vi "DB Message Loop.vi"(8 "error in (no error)":errorcluster, 11 "Message Queues":T1) -> (0 "error out":errorcluster)   [LabVIEW 2026]
uses:
  support/Message Queue/All Message Queues.ctl
  support/Message Queue/Message Cluster.ctl
  <vilib>/addons/database/Connection.llb/Conn ObjectReference.ctl
  controls/Telemetry_Data_Type.ctl
  controls/Channels.ctl
  controls/Error_Payload.ctl
  <vilib>/addons/database/Connection.llb/DB Tools Open Connec (String).vi
  <vilib>/addons/database/Connection.llb/Conn Execute.vi
  <vilib>/addons/database/Recordset.llb/Rec Destroy - Connection.vi
  <vilib>/Utility/error.llb/Error Cluster From Error Code.vi
  <vilib>/ErrorRing/Error Ring.xnode
  <vilib>/addons/database/NI_Database_API.lvlib
  support/Message Queue/Message Queue.lvlib
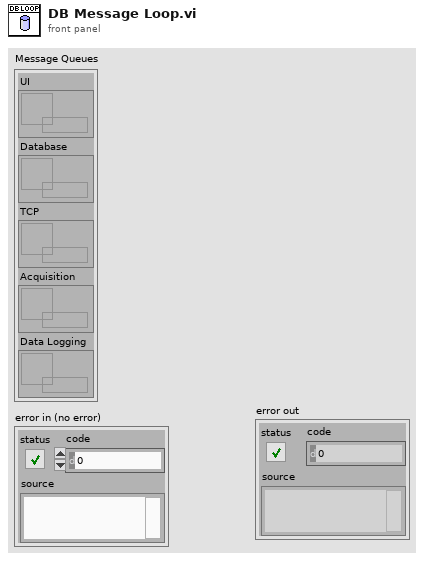
[diagram p1: front panel]
types:
  T1 = typedef "Message Queue.lvlib/All Message Queues.ctl" = cluster{"UI":refnum<queue>, "Database":refnum<queue>, "TCP":refnum<queue>, "Acquisition":refnum<queue>, "Data Logging":refnum<queue>}
  T2 = typedef "Error_Payload.ctl" = cluster{"status":bool, "error_code":i32, "description":string, "source_loop":string}
  T3 = typedef "NI_Database_API.lvlib/Conn ObjectReference.ctl" = refnum<k1>
  T4 = typedef "Telemetry_Data_Type.ctl" = cluster{"asset_id":i32, "channels":T5, "frame_id":i32}
  T5 = typedef "Channels.ctl" = cluster{"channel_id":dbl, "peak_frequency":dbl, "rms_acceleration":dbl, "health_score":dbl}[]
  T6 = typedef "NI_Database_API.lvlib/Rec ObjectReference.ctl" = refnum<k1>
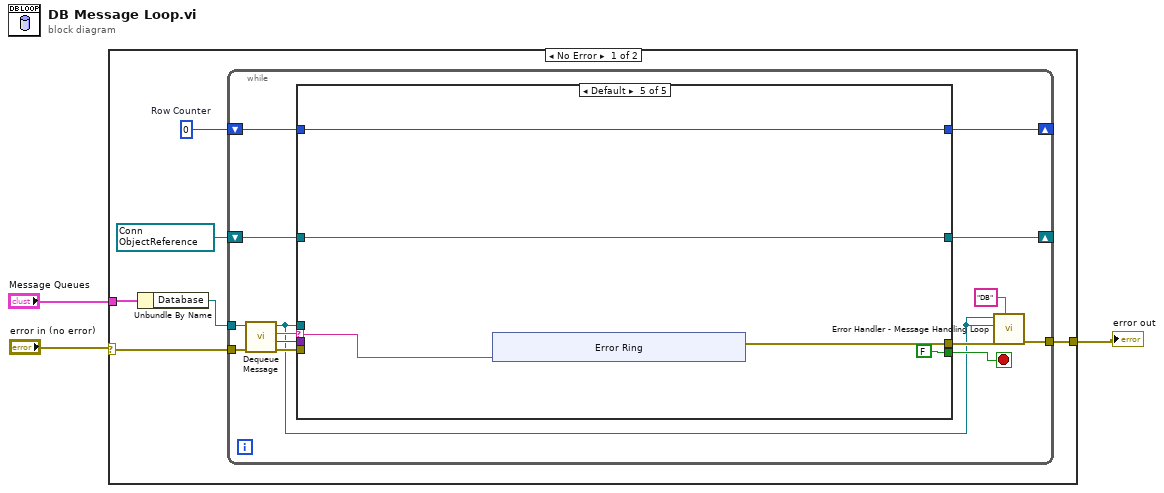
[diagram p0: block diagram]
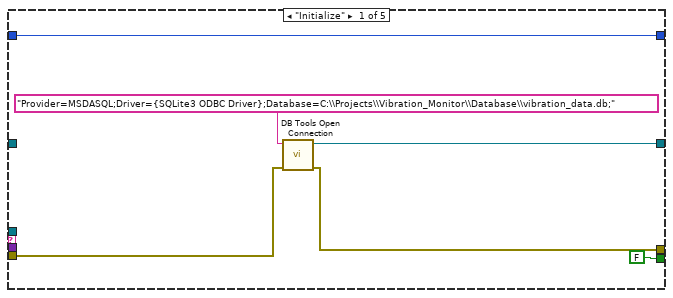
[diagram p2: hidden frame]
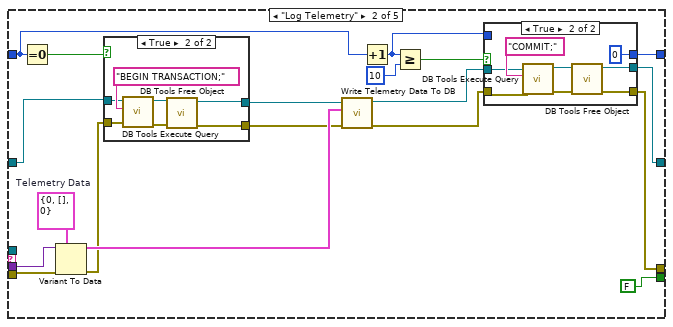
[diagram p3: hidden frame]
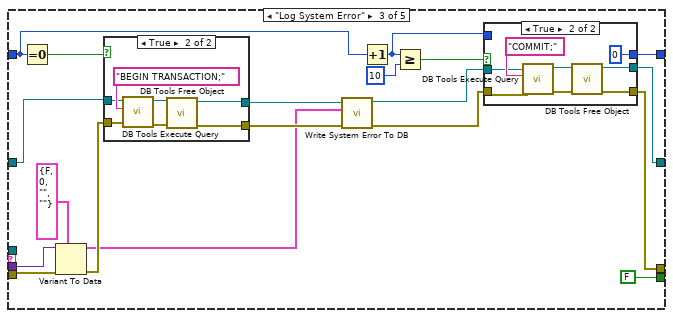
[diagram p6: hidden frame]
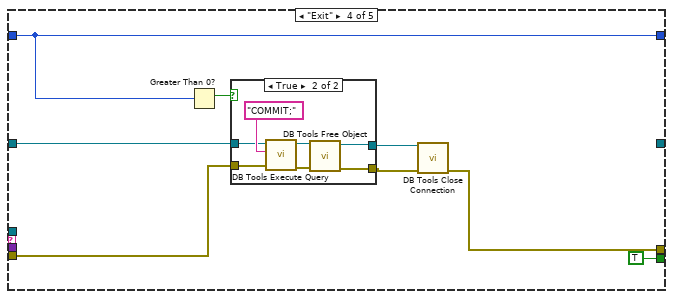
[diagram p9: hidden frame]
diagram:
  n1 = case shown="No Error" "error in (no error)" {
    selector: "error in (no error)" -> [w6 w137]
    tunnel: [w7 w137] -> w3
    tunnel: "Message Queues" -> [w5 _]
    frame No Error {
      w9 = T3 refnum items=["Connection"] ("connection reference")
      w8 = 0  # Row Counter
      n2 = Unbundle By Name(w5) -> ("Database"=w4:refnum<queue>)
      n3 = while {
        tunnel: w6 -> [w23]
        tunnel: [w18] -> w7
        shift-right: [w16] -> _
        shift-left: w9 -> [w15]
        shift-right: [w13] -> _
        shift-left: w8 -> [w14]
        tunnel: w4 -> [w12]
        stop <- w20 stop-if-true
        n4 = call "Dequeue Message.vi"("error in (no error)"=w23, "Message Queue"=w12) -> ("error out"=w21:errorcluster, "Message Data"=w17:variant, "Message"=w22:string, "dup Message Queue"=w11:refnum<queue>)  [unwired: 6 in]
        n5 = case shown="Default" w22 {
          selector: w22 -> [_ _ _ _ w128]
          tunnel: w11 -> [_ _ _ _ _]
          tunnel: w21 -> [w24 w47 w86 w108 _]
          tunnel: [FALSE FALSE FALSE TRUE FALSE] -> w20
          tunnel: [w27 w31 w72 w115 w127] -> w19
          tunnel: w17 -> [_ w46 w85 _ _]
          tunnel: [w26 w33 w74 _ w126] -> w16
          tunnel: w15 -> [_ w37 w78 w111 w126]
          tunnel: w14 -> [w25 w39 w80 w113 w125]
          tunnel: [w25 w40 w81 w113 w125] -> w13
          frame "Initialize" {
            n6 = call-poly <vilib>:"DB Tools Open Connection.vi"("error in (no error)"=w24, "connection information"="Provider=MSDASQL;Driver={SQLite3 ODBC Driver};Database=C:\\Projects\\Vibration_Monitor\\Database\\vibration_data.db;") -> ("error out"=w27:errorcluster, "connection reference"=w26:T3)  [unwired: 6 in]
          }
          frame "Log Telemetry" {
            w45 = T4 {"asset_id"=0, "channels"=[], "frame_id"=0}  # Telemetry Data
            n7 = Equal To 0?(x=w39) -> (x = 0?=w43:bool)
            n8 = Variant To Data(error in=w47, type=w45, Variant=w46) -> (data=w44:T4, error out=w30:errorcluster)
            n9 = case shown="True" w43 {
              tunnel: w30 -> [w61 w66]
              tunnel: [w61 w64] -> w36
              tunnel: w37 -> [w60 w63]
              tunnel: [w60 w62] -> w35
              frame False {
              }
              frame True {
                n10 = call-poly <vilib>:"DB Tools Execute Query.vi"("error in (no error)"=w66, "SQL query"="BEGIN TRANSACTION;" ("Message"), "connection reference"=w63) -> ("error out"=w65:errorcluster, "recordset reference"=w68:T6)  [unwired: 5 in]
                n11 = call-poly <vilib>:"DB Tools Free Object.vi"("error in (no error)"=w65, "recordset reference"=w68) -> ("error out"=w64:errorcluster, "connection reference"=w62:T3)  [unwired: 8 in]
              }
            }
            n12 = call "Write Telemetry Data To DB.vi"("error in (no error)"=w36, "Telemetry Data"=w44, "Refnum in"=w35) -> ("error out"=w32:errorcluster, "Refnum out"=w34:T3)  [unwired: 7 in]
            n13 = Increment(x=w39) -> (x+1=w38:i32)
            n14 = Greater Or Equal?(x=w38, y=10) -> (x >= y?=w41:bool)
            n15 = case shown="True" w41 {
              tunnel: [w51 0] -> w40
              tunnel: w38 -> [w51 _]
              tunnel: w34 -> [w50 w55]
              tunnel: [w50 w54] -> w33
              tunnel: w32 -> [w49 w53]
              tunnel: [w49 w52] -> w31
              frame False {
              }
              frame True {
                n16 = call-poly <vilib>:"DB Tools Execute Query.vi"("error in (no error)"=w53, "SQL query"="COMMIT;" ("Message"), "connection reference"=w55) -> ("error out"=w57:errorcluster, "recordset reference"=w56:T6)  [unwired: 5 in]
                n17 = call-poly <vilib>:"DB Tools Free Object.vi"("error in (no error)"=w57, "recordset reference"=w56) -> ("error out"=w52:errorcluster, "connection reference"=w54:T3)  [unwired: 8 in]
              }
            }
          }
          frame "Log System Error" {
            n18 = Equal To 0?(x=w80) -> (x = 0?=w84:bool)
            n19 = Variant To Data(error in=w86, type=T2 {"status"=FALSE, "error_code"=0, "description"="", "source_loop"=""} ("error constant"), Variant=w85) -> (data=w69:T2, error out=w71:errorcluster)
            n20 = case shown="True" w84 {
              tunnel: w71 -> [w100 w105]
              tunnel: [w100 w103] -> w77
              tunnel: w78 -> [w99 w102]
              tunnel: [w99 w101] -> w76
              frame False {
              }
              frame True {
                n21 = call-poly <vilib>:"DB Tools Execute Query.vi"("error in (no error)"=w105, "SQL query"="BEGIN TRANSACTION;" ("Message"), "connection reference"=w102) -> ("error out"=w104:errorcluster, "recordset reference"=w107:T6)  [unwired: 5 in]
                n22 = call-poly <vilib>:"DB Tools Free Object.vi"("error in (no error)"=w104, "recordset reference"=w107) -> ("error out"=w103:errorcluster, "connection reference"=w101:T3)  [unwired: 8 in]
              }
            }
            n23 = call "Write System Error To DB.vi"("error in (no error)"=w77, "Error_Payload"=w69, "Refnum in"=w76) -> ("error out"=w73:errorcluster, "Refnum out"=w75:T3)  [unwired: 7 in]
            n24 = Increment(x=w80) -> (x+1=w79:i32)
            n25 = Greater Or Equal?(x=w79, y=10) -> (x >= y?=w82:bool)
            n26 = case shown="True" w82 {
              tunnel: [w90 0] -> w81
              tunnel: w79 -> [w90 _]
              tunnel: w75 -> [w89 w94]
              tunnel: [w89 w93] -> w74
              tunnel: w73 -> [w88 w92]
              tunnel: [w88 w91] -> w72
              frame False {
              }
              frame True {
                n27 = call-poly <vilib>:"DB Tools Execute Query.vi"("error in (no error)"=w92, "SQL query"="COMMIT;" ("Message"), "connection reference"=w94) -> ("error out"=w96:errorcluster, "recordset reference"=w95:T6)  [unwired: 5 in]
                n28 = call-poly <vilib>:"DB Tools Free Object.vi"("error in (no error)"=w96, "recordset reference"=w95) -> ("error out"=w91:errorcluster, "connection reference"=w93:T3)  [unwired: 8 in]
              }
            }
          }
          frame "Exit" {
            n29 = Greater Than 0?(x=w113) -> (x > 0?=w112:bool)
            n30 = case shown="True" w112 {
              tunnel: w108 -> [w117 w122]
              tunnel: [w117 w119] -> w110
              tunnel: w111 -> [w116 w121]
              tunnel: [w116 w120] -> w109
              frame False {
              }
              frame True {
                n31 = call-poly <vilib>:"DB Tools Execute Query.vi"("error in (no error)"=w122, "SQL query"="COMMIT;" ("Message"), "connection reference"=w121) -> ("error out"=w118:errorcluster, "recordset reference"=w124:T6)  [unwired: 5 in]
                n32 = call-poly <vilib>:"DB Tools Free Object.vi"("error in (no error)"=w118, "recordset reference"=w124) -> ("error out"=w119:errorcluster, "connection reference"=w120:T3)  [unwired: 8 in]
              }
            }
            n33 = call <vilib>:"DB Tools Close Connection.vi"("error in (no error)"=w110, "connection reference"=w109) -> ("error out"=w115:errorcluster)  [unwired: 5 in]
          }
          frame Default {
            n34 = xnode "Error Ring"("parameter 0"=w128) -> ("error out"=w127:errorcluster)
          }
        }
        n35 = call "Error Handler - Message Handling Loop.vi"("Loop Name"="DB", "error in (no error)"=w19, "Database"=w11, "Message Queue"=w11) -> ("dup error in"=w18:errorcluster)  [unwired: 6 in, 1 out]
      }
    }
    frame Error {
    }
  }
  "error out" <- w3
